vi "thermal PRF check by PID.vi"(0 "meas_setting":T2={"measSetId"=6949, "measSetComments"="Orchid", "probeId"=141.0, "beamstyleIndex"=0, "txFrequencyHz"=3636400.0, "focusRangeCm"=8.0, "maxTxVoltageVolt"=100.0, "ceilTxVoltageVolt"=80.0, "profTxVoltageVolt"=62.0, "totalVoltagePt"=20, "numMeasVoltage"=12, "numTxElements"=118, "txpgWaveformStyle"=2, "numTxCycles"=4.0, "elevAperIndex"=0, "zStartDistCm"=1.5, "zMeasNum"=80, "IsTxAperModulationEn"=0, "DTxFreqIndex"=0, "VTxIndex"=0, "IsCPAEn"=0, "SysPulserSelA"=0, "TxPulseRleA"=""} {"zStartDistCm" format="%.2f"; "numTxCycles" format="%.1f"; "profTxVoltageVolt" format="%#_1g"; "ceilTxVoltageVolt" format="%.2f"; "maxTxVoltageVolt" format="%.2f"; "focusRangeCm" format="%.1f"; "txFrequencyHz" format="%.2f"}, 1 "PRF":dbl format="%.2f", 2 "Measurement Type":enum32{"Volt", "SA"}(radio), 5 "TCP from Orchid in":refnum<k5>, 9 "tcp time out":dbl format="%.2f", 11 "voltage":dbl format="%.2f", 12 "Comment(SN)":string) -> (4 "PRF":dbl format="%#.2f", 10 "Command \nVerify":bool, 15 "Error(Volt & PRF)":bool)   [LabVIEW 2016]
uses:
  type def/measSetting.ctl
  user/GrobaLimitVoltage.vi
  Thermal_type.vi
  <vilib>/Instr/_visa.llb/VISA Configure Serial Port (Instr).vi
  Instance          12 30Saved   thermal PRF&Volt check .vi
  Instance          18 30Saved   thermal PRF&Volt check .vi
panel:
  out "error out 4":errorcluster
  out "error out 3":errorcluster
  in  "취소 버튼":bool
  out "경과시간(S)":string caption="경과 시간 텍스트"
  out "TempRise":dbl format="%.2f"
  out "Probe":dbl format="%.2f"
  out "Ambient":dbl format="%.2f"
  out "웨이브폼 차트":dbl(graph)
  out "경과시간":dbl caption="경과 시간(초)" format="%#.1g"
  out "Finish Time":string="7/29/2002  5:00 PM"
  out "Target  Temp.":i32
  out "Ambient":dbl
  out "Transducer":dbl
  out "error out 2":errorcluster
  out "Initial PRF":dbl format="%.2f"
  out "Current Voltage":dbl format="%.2f"
  out "Output Limit Voltage":i16
  out "Start Time":string="7/29/2002  5:00 PM"
  in  "stop 3":bool
  in  "meas_temparature_result":T1={"probeId"=10.0, "comments"="4C1 WCS", "tempSSId"=2, "measDate"="", "measSetNum"=1, "roomTempC"=0.0, "pulseVoltage"=80.0, "temperatureC"=0.0, "numTxCycles"=3.0, "numTxElements"=22, "txFrequencyHz"=3636400.0, "elevAperIndex"=0, "isTxAperModulationEn"=0, "txpgWaveformStyle"=0, "pulseRepetRate"=610.0, "scanRange"=0.0, "tempSetId"=0, "IsSCW"=0, "VTxIndex"=0} {"temperatureC" format="%.2f"; "scanRange" format="%.2f"; "pulseRepetRate" format="%.6f"; "roomTempC" format="%.2f"; "numTxCycles" format="%#_1f"}
  out "Result":string
  in  "file path":path=path "C:/temp log data/TempResultData"
  out "Waveform Chart":cluster{dbl, dbl, i32, i32}(graph)
  out "error out":errorcluster
  # "To find PRF by PID"
  # "Cooling"
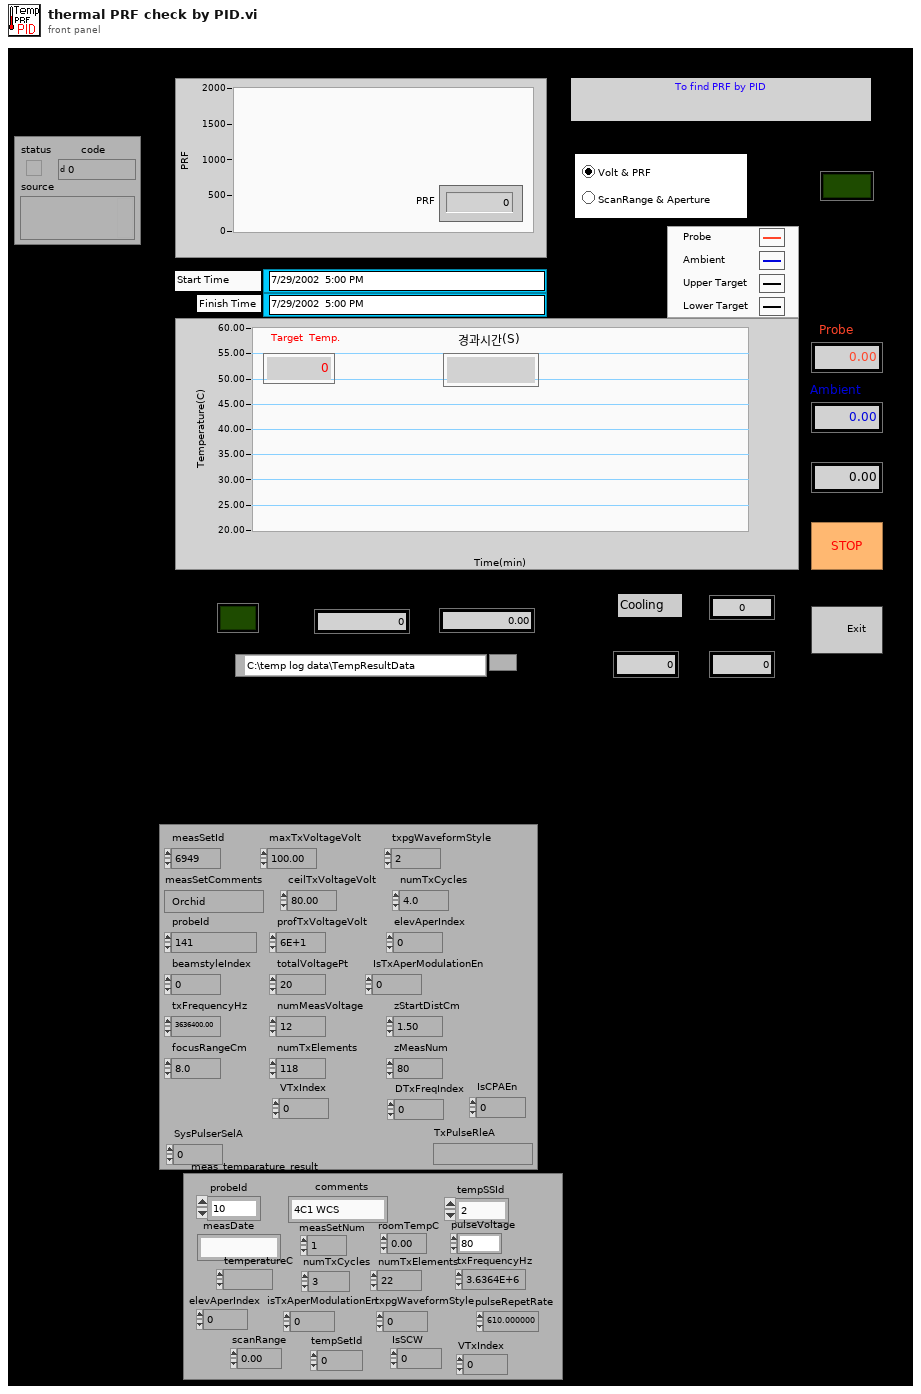
[diagram p1: front panel]
types:
  T1 = cluster{"probeId":sgl, "comments":string, "tempSSId":i16, "measDate":string, "measSetNum":i16, "roomTempC":sgl, "pulseVoltage":dbl, "temperatureC":ext, "numTxCycles":dbl, "numTxElements":i16, "txFrequencyHz":dbl, "elevAperIndex":i16, "isTxAperModulationEn":i16, "txpgWaveformStyle":i16, "pulseRepetRate":dbl, "scanRange":dbl, "tempSetId":i16, "IsSCW":i16, "VTxIndex":i16}
  T2 = typedef "measSetting.ctl" = cluster{"measSetId":i32, "measSetComments":string, "probeId":sgl, "beamstyleIndex":i16, "txFrequencyHz":sgl, "focusRangeCm":sgl, "maxTxVoltageVolt":sgl, "ceilTxVoltageVolt":sgl, "profTxVoltageVolt":dbl, "totalVoltagePt":i8, "numMeasVoltage":i8, "numTxElements":i16, "txpgWaveformStyle":i8, "numTxCycles":sgl, "elevAperIndex":i8, "zStartDistCm":sgl, "zMeasNum":i8, "IsTxAperModulationEn":i8, "DTxFreqIndex":i16, "VTxIndex":i8, "IsCPAEn":i16, "SysPulserSelA":i16, "TxPulseRleA":string}
  T3 = enum16{"open", "open or create", "create or replace", "create", "open (read only)"}
  T4 = cluster{"Output probe":dbl, "Output ambient":dbl, i32, i32}
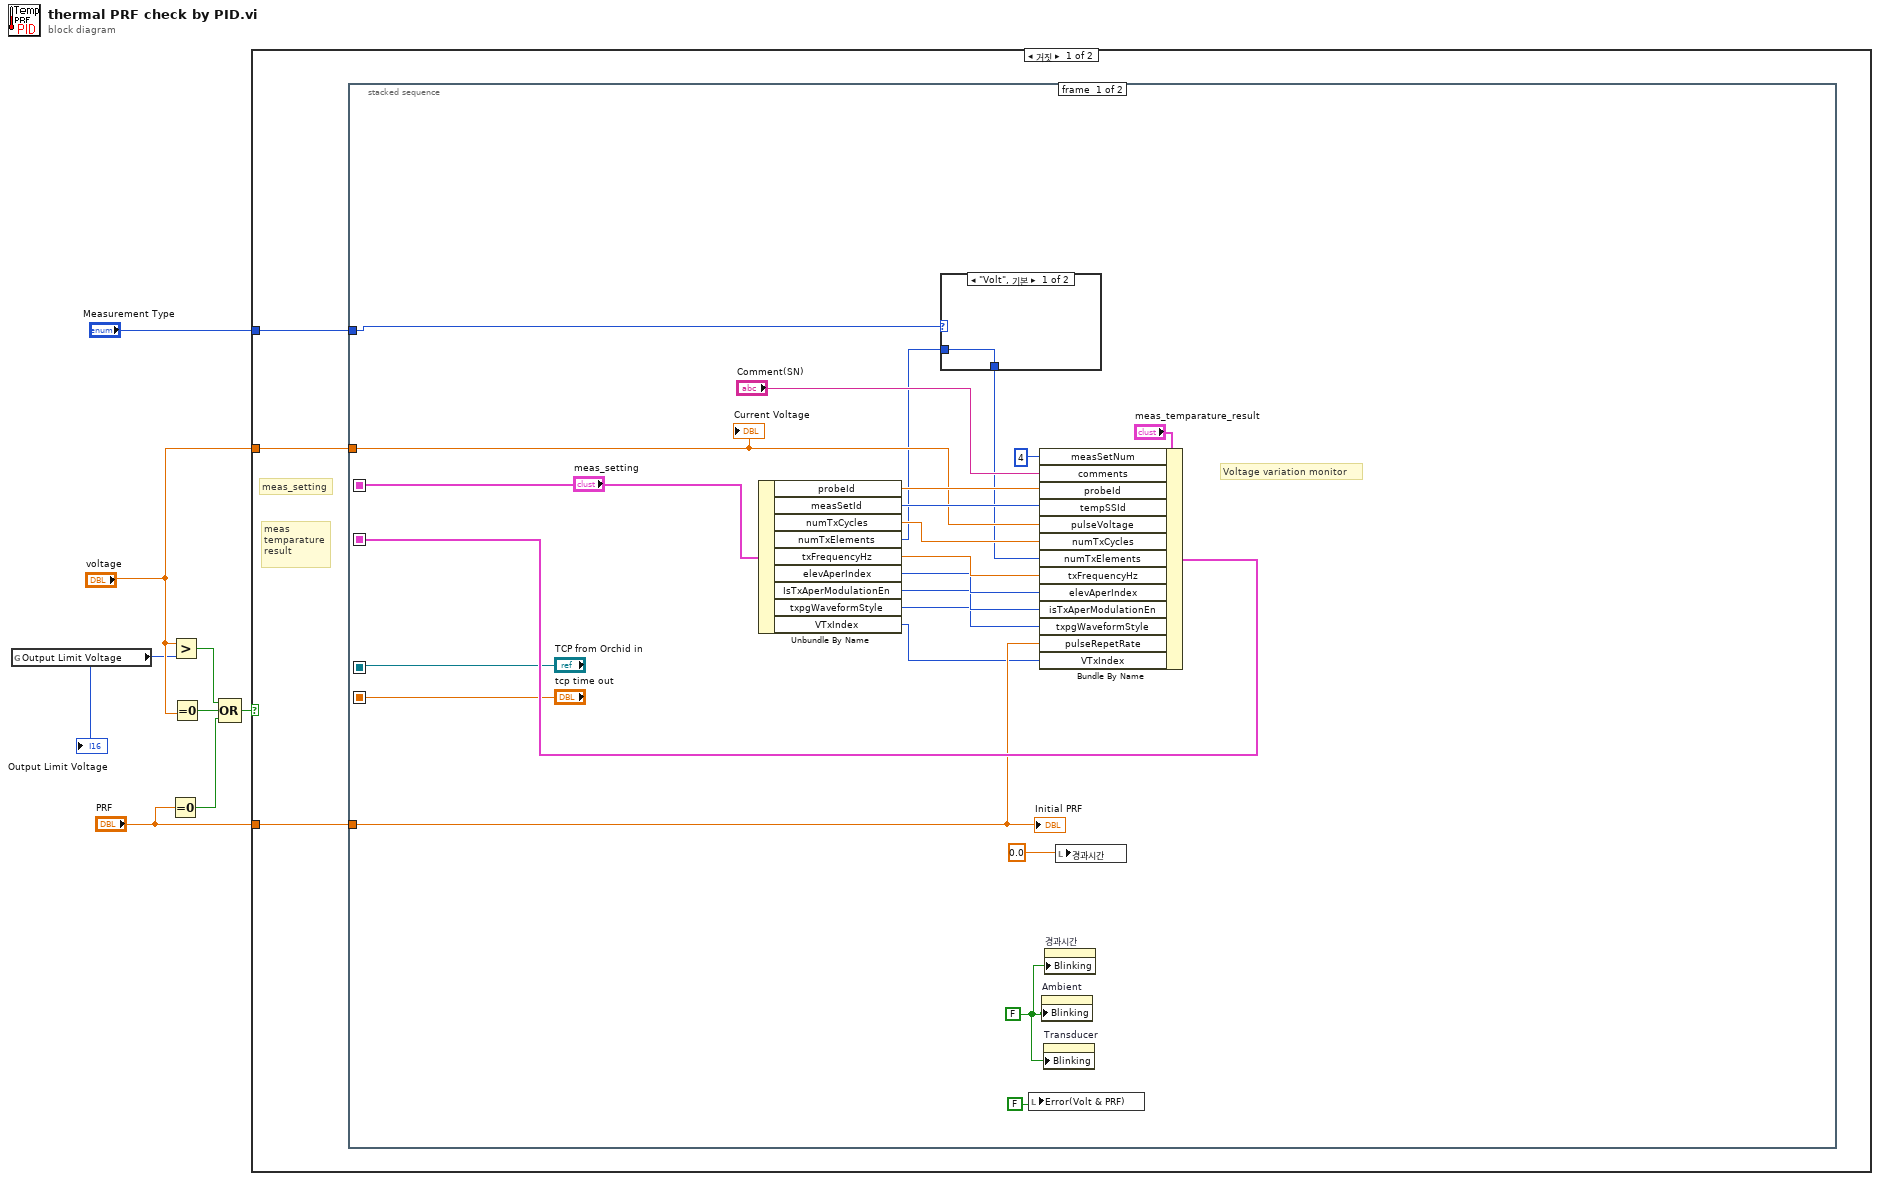
[diagram p0: block diagram]
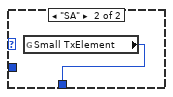
[diagram p2: hidden frame]
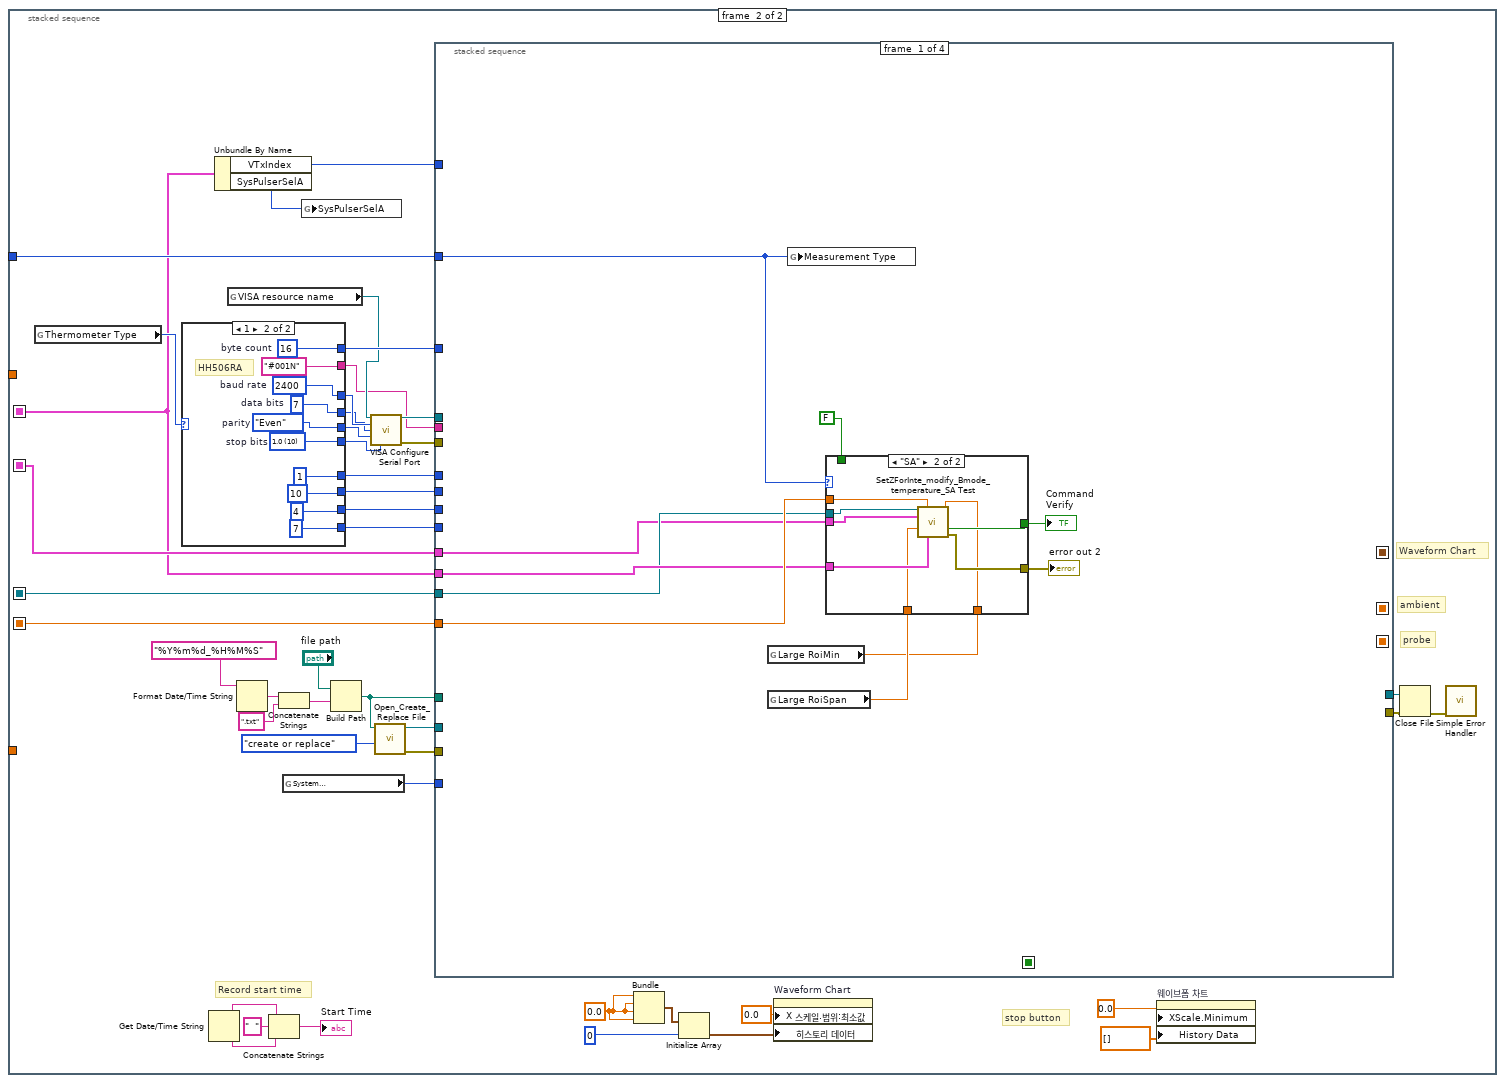
[diagram p3: hidden frame]
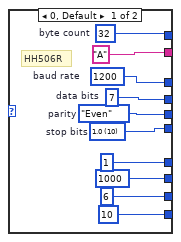
[diagram p4: hidden frame]
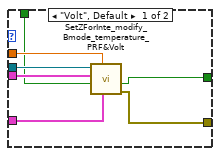
[diagram p5: hidden frame]
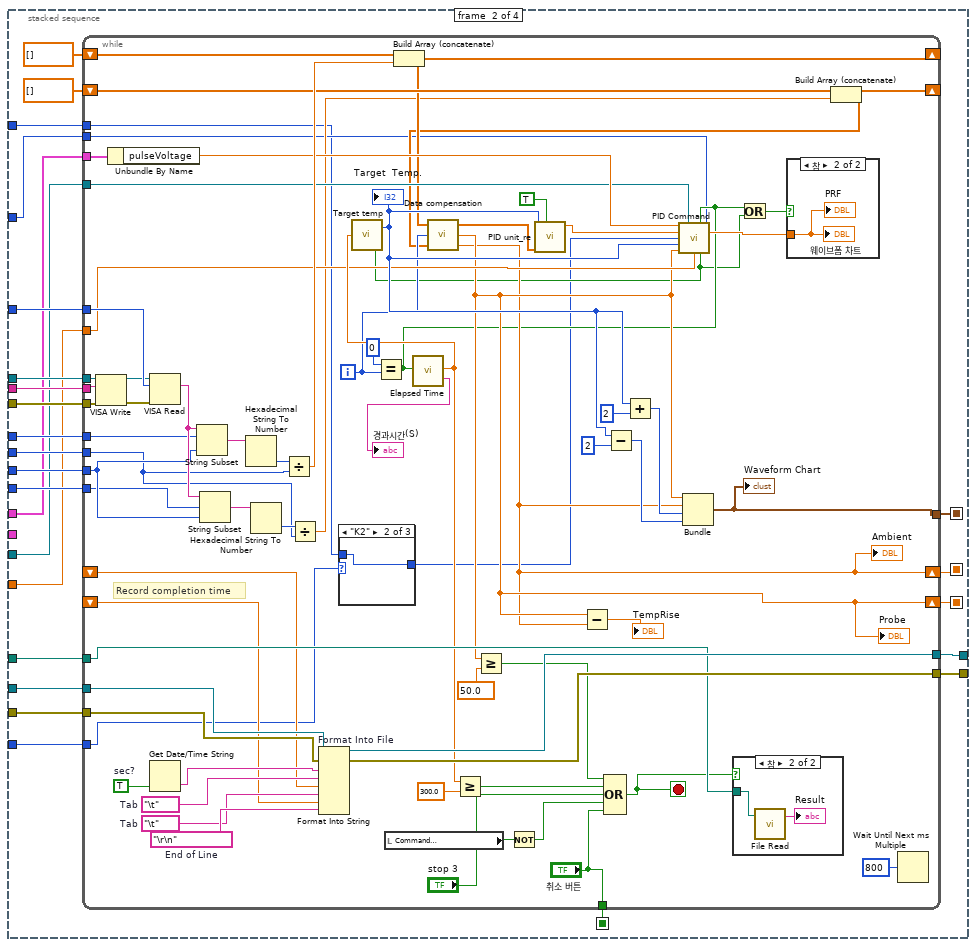
[diagram p6: hidden frame]
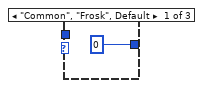
[diagram p7: hidden frame]
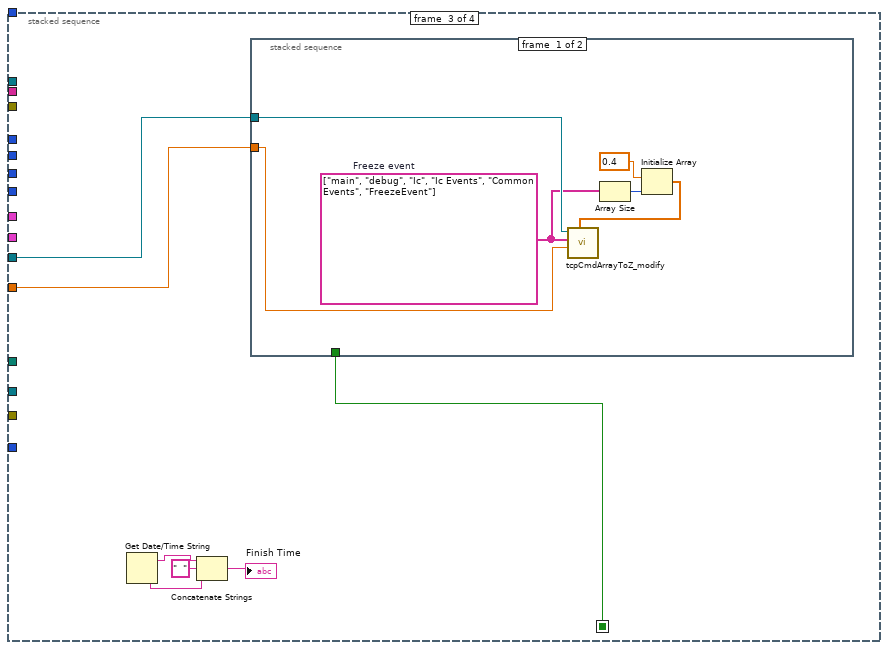
[diagram p11: hidden frame]
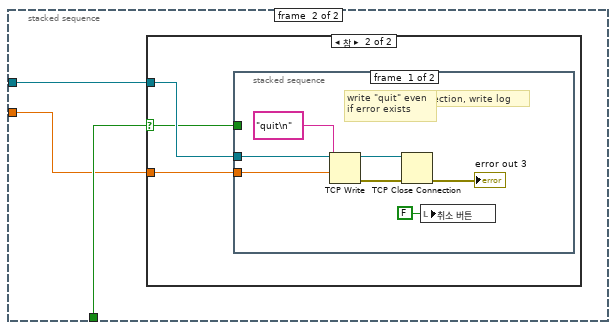
[diagram p12: hidden frame]
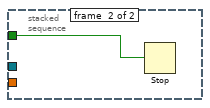
[diagram p14: hidden frame]
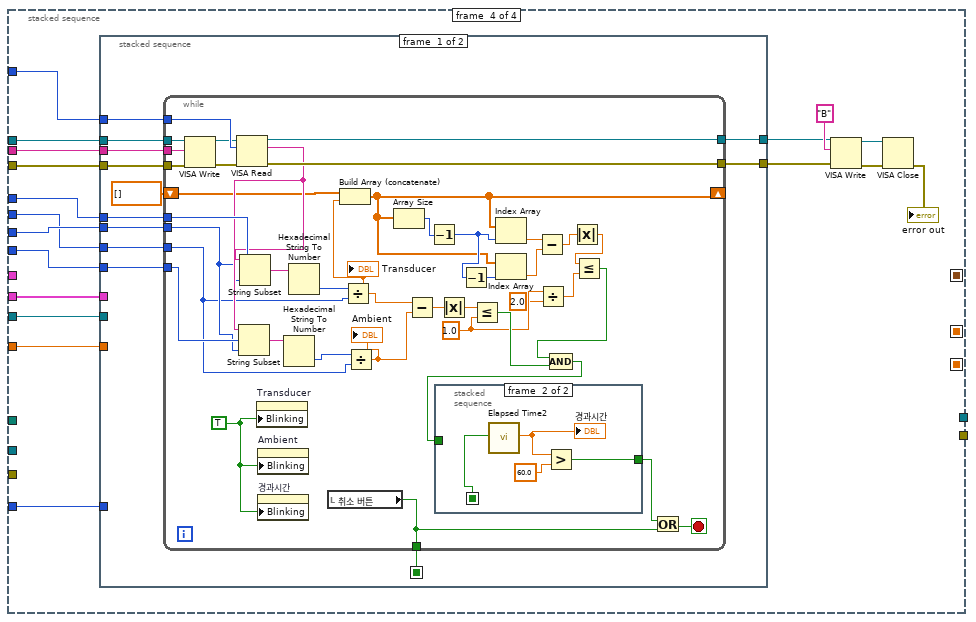
[diagram p15: hidden frame]
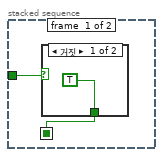
[diagram p16: hidden frame]
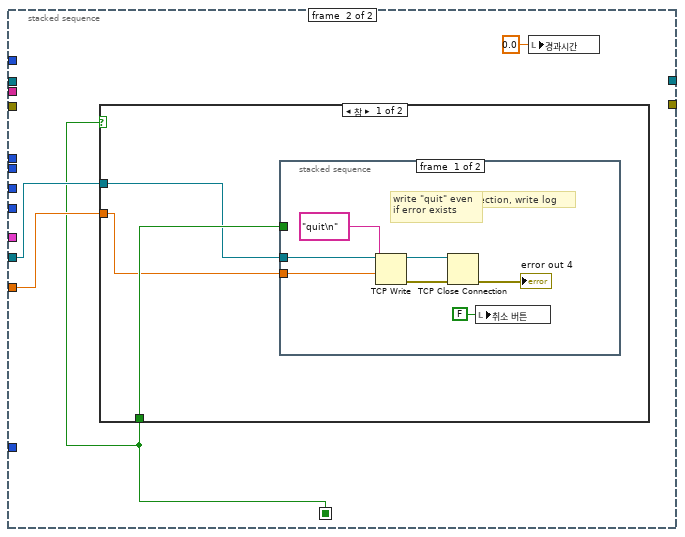
[diagram p18: hidden frame]
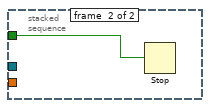
[diagram p19: hidden frame]
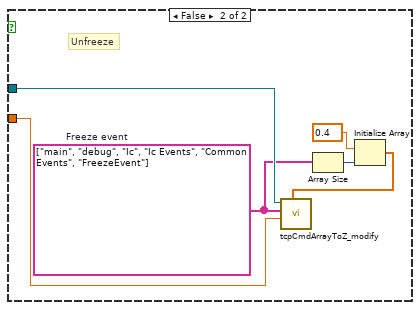
[diagram p20: hidden frame]
diagram:
  n1 = global read "GrobaLimitVoltage.vi" "Output Limit Voltage"() -> (w7:i16)
  "Output Limit Voltage" <- w7
  n2 = Equal To 0?(x="PRF") -> (x = 0?=w2:bool)
  n3 = Greater?(x="voltage", y=w7) -> (0:w6:bool)
  n4 = Equal To 0?(x="voltage") -> (x = 0?=w5:bool)
  n5 = Compound Arithmetic op=OR(w6, w5, w2) -> (w4:bool)
  n6 = case shown="거짓" w4 {
    tunnel: "voltage" -> [w11 _]
    tunnel: "PRF" -> [w10 _]
    tunnel: "Measurement Type" -> [w9 _]
    frame False {
      # "meas\ntemparature\nresult"
      # "meas_setting"
      n7 = stacked-sequence {
        seq-local: ["meas_setting" _] -> [_ w38]
        seq-local: [w24 _] -> [_ w69]
        seq-local: ["TCP from Orchid in" _] -> [_ w68]
        seq-local: ["tcp time out" _] -> [_ w67]
        tunnel: w11 -> [w22 _]
        tunnel: w10 -> [w21 _]
        tunnel: w9 -> [w15 w41]
        frame #0 {
          w17 = FALSE ("점멸")
          # "Voltage variation monitor"
          n8 = Unbundle By Name("meas_setting") -> ("probeId"=w31:sgl, "measSetId"=w30:i32, "numTxCycles"=w29:sgl, "numTxElements"=w13:i16, "txFrequencyHz"=w28:sgl, "elevAperIndex"=w27:i8, "IsTxAperModulationEn"=w26:i8, "txpgWaveformStyle"=w25:i8, "VTxIndex"=w12:i8)
          n9 = case shown="\"Volt\", 기본" w15 {
            tunnel: [w35 w36] -> w14
            tunnel: w13 -> [w35 _]
            frame "Volt", Default {
            }
            frame "SA" {
              n10 = global read "Thermal_type.vi" "Small TxElement"() -> (w36:i32)
            }
          }
          n11 = local write "Error(Volt & PRF)"(FALSE) -> ()
          n12 = Bundle By Name(cluster="meas_temparature_result", "measSetNum"=i16 4, "comments"="Comment(SN)", "probeId"=w31, "tempSSId"=w30, "pulseVoltage"=w22, "numTxCycles"=w29, "numTxElements"=w14, "txFrequencyHz"=w28, "elevAperIndex"=w27, "isTxAperModulationEn"=w26, "txpgWaveformStyle"=w25, "pulseRepetRate"=w21, "VTxIndex"=w12) -> (w24:T1)
          n13 = property on="Ambient" class="DigNum (엄격한)"("Blinking"=w17) -> ()  [unwired: 2 in, 2 out]
          n14 = property on="Transducer" class="DigNum (엄격한)"("Blinking"=w17) -> ()  [unwired: 2 in, 2 out]
          n15 = property on="경과시간" class="DigNum (엄격한)"("Blinking"=w17) -> ()  [unwired: 2 in, 2 out]
          n16 = local write "경과시간"(0.0 ("Elapsed Time (s)")) -> ()
          "Current Voltage" <- w22
          "Initial PRF" <- w21
        }
        frame #1 {
          w44 = 0.0
          # "Record start time"
          # "Waveform Chart"
          # "ambient"
          # "probe"
          # "stop button"
          n17 = global read "Thermal_type.vi" "Thermometer Type"() -> (w59:u16)
          n18 = case shown="1" w59 {
            tunnel: [w91 w100] -> w57
            tunnel: [w90 w99] -> w56
            tunnel: [w89 w98] -> w55
            tunnel: ["A" ("write buffer (\"\")") "#001N" ("write buffer (\"\")")] -> w46
            tunnel: [w87 w97] -> w54
            tunnel: [10 ("offset (0)") 7 ("offset (0)")] -> w51
            tunnel: [6 ("length (rest)") 4 ("length (rest)")] -> w52
            tunnel: [u32 1000 ("y") u32 10 ("y")] -> w50
            tunnel: [1 ("offset (0)") 1 ("offset (0)")] -> w53
            tunnel: [w82 w92] -> w58
            frame 0, Default {
              w82 = u32 32  # byte count
              w87 = u16 10 items=["1.0"=10, "1.5"=15, "2.0"=20]  # stop bits
              w89 = enum16{"None", "Odd", "Even", "Mark", "Space"}."Even"  # parity
              w90 = u16 7  # data bits
              w91 = u32 1200  # baud rate
              # "HH506R"
            }
            frame 1 {
              w92 = u32 16  # byte count
              w97 = u16 10 items=["1.0"=10, "1.5"=15, "2.0"=20]  # stop bits
              w98 = enum16{"None", "Odd", "Even", "Mark", "Space"}."Even"  # parity
              w99 = u16 7  # data bits
              w100 = u32 2400  # baud rate
              # "HH506RA"
            }
          }
          n19 = Get Date/Time String() -> (date string=w65:string, time string=w63:string)  [unwired: 3 in]
          n20 = Unbundle By Name(w38) -> ("VTxIndex"=w40:i8, "SysPulserSelA"=w37:i16)
          n21 = global read "Thermal_type.vi" "VISA resource name"() -> (w49:refnum<visa-resource-name>)
          n22 = Format Date/Time String(time format string (%c)="%Y%m%d_%H%M%S") -> (date/time string=w62:string)  [unwired: 2 in]
          n23 = Concatenate Strings(w65, "  ", w63) -> (→"Start Time":string)
          n24 = Concatenate Strings(w62, ".txt" ("string")) -> (w70:string)
          n25 = global read "Thermal_type.vi" "System \nSelection"() -> (w39:enum32{"Common", "Frosk", "Griffin", "K2"})
          n26 = global write "Thermal_type.vi" "SysPulserSelA"(w37) -> ()
          n27 = Build Path(base path="file path", name or relative path=w70) -> (appended path=w71:path)
          n28 = call-poly "VISA Configure Serial Port"("VISA resource name"=w49, "baud rate (9600)"=w57, "data bits (8)"=w56, "parity (0:none)"=w55, "stop bits (10: 1 bit)"=w54) -> ("VISA resource name out"=w48:refnum<visa-resource-name>, "error out"=w47:errorcluster)  [unwired: 9 in]
          n29 = call <vilib>:"Open_Create_Replace File.vi"("function (open:0)"=T3."create or replace", "file path"=w71) -> ("error out"=w80:errorcluster, "refnum"=w81:refnum<file>)  [unwired: 6 in, 2 out]
          n30 = stacked-sequence {
            seq-local: [_ w146 _ _] -> [_ _ _ _]
            seq-local: [_ w145 _ _] -> [_ _ _ _]
            seq-local: [_ w144 _ _] -> [_ _ _ _]
            seq-local: [_ w127 _ _] -> [_ _ w229 _]
            tunnel: w81 -> [_ w151 _ _]
            tunnel: w80 -> [_ w150 _ _]
            tunnel: [_ w149 _ _] -> w78
            tunnel: [_ w148 _ _] -> w76
            tunnel: w71 -> [_ w147 _ _]
            tunnel: w69 -> [w108 w132 _ _]
            tunnel: w68 -> [w109 w135 w231 w267]
            tunnel: w67 -> [w111 w134 w230 w266]
            tunnel: w38 -> [w110 _ _ w257]
            tunnel: w58 -> [_ w143 _ w262]
            tunnel: w53 -> [_ w142 _ w265]
            tunnel: w52 -> [_ w141 _ w264]
            tunnel: w51 -> [_ w140 _ w258]
            tunnel: w50 -> [_ w139 _ w263]
            tunnel: w48 -> [_ w138 _ w261]
            tunnel: w47 -> [_ w137 _ w260]
            tunnel: w46 -> [_ w136 _ w259]
            tunnel: w41 -> [w105 w128 _ _]
            tunnel: w40 -> [_ w130 _ _]
            tunnel: w39 -> [_ w129 _ w256]
            frame #0 {
              n31 = global read "Thermal_type.vi" "Large RoiMin"() -> (w103:dbl)
              n32 = global read "Thermal_type.vi" "Large RoiSpan"() -> (w104:dbl)
              n33 = global write "Thermal_type.vi" "Measurement Type"(w105) -> ()
              n34 = case shown="\"SA\"" w105 {
                tunnel: w111 -> [w118 w123]
                tunnel: w110 -> [w117 w125]
                tunnel: w109 -> [w116 w126]
                tunnel: w108 -> [w115 w124]
                tunnel: [w114 w122] -> w107
                tunnel: [w113 w121] -> w106
                tunnel: w104 -> [_ w120]
                tunnel: w103 -> [_ w119]
                tunnel: FALSE ("CW") -> [w112 _]
                frame "Volt", Default {
                  n35 = call "SetZForInte_modify_Bmode_temperature_PRF&Volt.vi"("meas_setting"=w117, "timeout (ms)"=w118, "CW"=w112, "meas_temparature_Input"=w115, "TCP from Orchid in"=w116) -> ("error out"=w113:errorcluster, "veri_P/F"=w114:bool)  [unwired: 3 in, 2 out]
                }
                frame "SA" {
                  n36 = call "SetZForInte_modify_Bmode_temperature_SA Test.vi"("TCP from Orchid in"=w126, "timeout (ms)"=w123, "RoiLaterMin"=w119, "meas_temparature_Input"=w124, "RoiLateralSpan"=w120, "meas_setting"=w125) -> ("veri_P/F"=w122:bool, "error out"=w121:errorcluster)  [unwired: 6 in, 2 out]
                }
              }
              "Command \nVerify" <- w107
              "error out 2" <- w106
            }
            frame #1 {
              n37 = while {
                shift-right: [w162] -> w146
                shift-left: _ -> [w203]
                shift-right: [w163] -> w145
                shift-left: _ -> [w190]
                tunnel: w151 -> [w219]
                tunnel: w150 -> [w218]
                tunnel: [w217] -> w148
                tunnel: [w216] -> w149
                tunnel: w147 -> [w212]
                tunnel: [w188] -> w144
                tunnel: w143 -> [w200]
                tunnel: w142 -> [w199]
                tunnel: w141 -> [w198]
                tunnel: w140 -> [w197]
                tunnel: w139 -> [w196]
                tunnel: w138 -> [w195]
                tunnel: w137 -> [w194]
                tunnel: w136 -> [w191]
                tunnel: w135 -> [w170]
                tunnel: w134 -> [w171]
                shift-right: [w168] -> _
                shift-left: dbl[] [] -> [w187]
                tunnel: w132 -> [w184]
                shift-right: [w165] -> _
                shift-left: dbl[] [] -> [w169]
                tunnel: w130 -> [w152]
                tunnel: w129 -> [w156]
                tunnel: w128 -> [w154]
                tunnel: ["취소 버튼"] -> w127
                i -> [w166]
                stop <- w210 stop-if-true
                w214 = "\t"  # Tab
                w215 = "\r\n"  # End of Line
                w220 = "\t"  # Tab
                w221 = TRUE  # sec?
                # "Record completion time"
                n38 = VISA Write(VISA resource name=w195, write buffer=w191, error in (no error)=w194) -> (VISA resource name out=w193:refnum<visa-resource-name>, error out=w192:errorcluster)  [unwired: 1 out]
                n39 = Unbundle By Name(w184) -> ("pulseVoltage"=w174:dbl)
                n40 = VISA Read(VISA resource name=w193, byte count=w200, error in (no error)=w192) -> (read buffer=w202:string)  [unwired: 3 out]
                n41 = Get Date/Time String(want seconds? (F)=w221) -> (time string=w213:string)  [unwired: 2 in, 1 out]
                n42 = String Subset(string=w202, offset (0)=w199, length (rest)=w198) -> (substring=w207:string)
                n43 = String Subset(string=w202, offset (0)=w197, length (rest)=w198) -> (substring=w205:string)
                n44 = Hexadecimal String To Number(string=w207) -> (number=w206:u32)  [unwired: 2 in, 1 out]
                n45 = Hexadecimal String To Number(string=w205) -> (number=w204:u32)  [unwired: 2 in, 1 out]
                n46 = Divide(x=w206, y=w196) -> (x/y=w175:dbl)
                n47 = Divide(x=w204, y=w196) -> (x/y=w164:dbl)
                n48 = Format Into String "Format Into File"(initial string=w219, error in=w218, w213, w220, w203, w214, w190, w215) -> (resulting string=w217:refnum<file>, error out=w216:errorcluster)  [unwired: 1 in]
                n49 = case shown="\"K2\"" w156 {
                  tunnel: [0 w224 w225] -> w155
                  tunnel: w152 -> [_ w224 w225]
                  frame "Common", "Frosk", Default {
                  }
                  frame "K2" {
                  }
                  frame "Griffin" {
                  }
                }
                n50 = Equal?(x=0, y=w166) -> (x = y?=w159:bool)
                n51 = local read "Command \nVerify"() -> (w186:bool)
                n52 = Build Array (concatenate)(w187, w175) -> (w168:dbl[])
                n53 = call "Elapsed Time"("Reset"=w159) -> ("Elapsed Time (s)"=w181:dbl, "Elapsed Time Text"=→"경과시간(S)":string)  [unwired: 11 in, 6 out]
                n54 = call "Target temp.vi"("elapsed time"=w181) -> ("Target temperature"=w172:i32, "control"=w158:bool)
                "Target  Temp." <- w172
                n55 = Greater Or Equal?(x=w181, y=300.0) -> (x >= y?=w182:bool)
                n56 = Not(x=w186) -> (.not. x?=w185:bool)
                n57 = Subtract(x=w172, y=2) -> (x-y=w176:i32)
                n58 = Add(x=w172, y=2) -> (x+y=w178:i32)
                n59 = Or(x=w159, y=w158) -> (x .or. y?=w160:bool)
                n60 = Build Array (concatenate)(w169, w164) -> (w165:dbl[])
                n61 = call "Data compensation.vi"("Input ambient"=w165, "Index"=w166, "Input probe"=w168) -> ("Output ambient"=w162:dbl, "Output probe"=w163:dbl, "Output probe array"=w167:dbl[])
                "Ambient" <- w162
                "Probe" <- w163
                n62 = Greater Or Equal?(x=w163, y=50.0) -> (x >= y?=w209:bool)
                n63 = call "PID unit_re.vi"("PID"=TRUE, "현재 온도"=w167, "Target 온도"=w172) -> ("적정 PRF"=w173:dbl)  [unwired: 6 in]
                n64 = Subtract(x=w163, y=w162) -> (x-y=→"TempRise":dbl)
                n65 = Compound Arithmetic op=OR(w209, w182, "stop 3", w185, "취소 버튼") -> (w210:bool)
                n66 = call "PID Command.vi"("PulseVoltage"=w174, "TCP from Orchid in"=w170, "Starting index"=w159, "Measurement Type"=w154, "적정 PRF"=w173, "VTxIndex"=w155, "Target temp"=w172, "Probe temp"=w163, "tcp time out"=w171, "Control enable"=w158) -> ("PRF"=w161:dbl)  [unwired: 5 in]
                n67 = Bundle("Output probe"=w163, "Output ambient"=w162, w178, w176) -> (w188:T4)  [unwired: 1 in]
                "Waveform Chart" <- w188
                n68 = case shown="참" w210 {
                  tunnel: w212 -> [_ w227]
                  frame False {
                  }
                  frame True {
                    n69 = call "File Read.vi"("file path"=w227) -> ("data"=→"Result":string)  [unwired: 3 in]
                  }
                }
                n70 = case shown="참" w160 {
                  tunnel: w161 -> [_ w226]
                  frame False {
                  }
                  frame True {
                    "웨이브폼 차트" <- w226
                    "PRF" <- w226
                  }
                }
                n71 = Wait Until Next ms Multiple(millisecond multiple=u32 800 ("milliseconds to wait")) -> ()  [unwired: 1 out]
              }
            }
            frame #2 {
              n72 = Get Date/Time String() -> (date string=w232:string, time string=w235:string)  [unwired: 3 in]
              n73 = Concatenate Strings(w232, "  ", w235) -> (→"Finish Time":string)
              n74 = stacked-sequence {
                tunnel: w231 -> [w241 w243]
                tunnel: w230 -> [w240 w242]
                tunnel: w229 -> [_ w244]
                frame #0 {
                  w237 = string[] ["main", "debug", "Ic", "Ic Events", "Common Events", "FreezeEvent"]  # Freeze event
                  n75 = Array Size(array=w237) -> (size(s)=w239:i32)
                  n76 = Initialize Array(0.4 ("element"), w239) -> (w236:dbl[])
                  n77 = call "tcpCmdArrayToZ_modify.vi"("Delay (sec)"=w236, "Timeout (ms)"=w240, "Command array"=w237, "connection ID in"=w241) -> ()  [unwired: 3 in, 5 out]
                }
                frame #1 {
                  n78 = case shown="참" w244 {
                    selector: w244 -> [_ w245]
                    tunnel: w243 -> [_ w247]
                    tunnel: w242 -> [_ w246]
                    frame False {
                    }
                    frame True {
                      n79 = stacked-sequence {
                        tunnel: w247 -> [w250 _]
                        tunnel: w246 -> [w249 _]
                        tunnel: w245 -> [_ w255]
                        frame #0 {
                          # "Close telnet connection, write log"
                          # "write \"quit\" even\nif error exists"
                          n80 = TCP Write(connection ID=w250, data in="quit\n", 9:w249) -> (connection ID out=w251:refnum<k5>, error out=w253:errorcluster)  [unwired: 1 in, 1 out]
                          n81 = TCP Close Connection(connection ID=w251, error in (no error)=w253) -> (error out=→"error out 3":errorcluster)  [unwired: 1 in, 1 out]
                          n82 = local write "취소 버튼"(FALSE ("취소 버튼")) -> ()
                        }
                        frame #1 {
                          n83 = Stop(stop? (T)=w255) -> ()
                        }
                      }
                    }
                  }
                }
              }
            }
            frame #3 {
              n84 = stacked-sequence {
                seq-local: [w274 _] -> [_ w333]
                tunnel: [w285 _] -> w269
                tunnel: [w284 _] -> w268
                tunnel: w267 -> [_ w335]
                tunnel: w266 -> [_ w334]
                tunnel: w265 -> [w283 _]
                tunnel: w264 -> [w282 _]
                tunnel: w263 -> [w281 _]
                tunnel: w262 -> [w280 _]
                tunnel: w261 -> [w279 _]
                tunnel: w260 -> [w278 _]
                tunnel: w259 -> [w277 _]
                tunnel: w258 -> [w276 _]
                tunnel: w257 -> [_ _]
                tunnel: w256 -> [_ _]
                frame #0 {
                  n85 = while {
                    tunnel: [w323] -> w285
                    tunnel: [w322] -> w284
                    tunnel: w283 -> [w321]
                    tunnel: w282 -> [w312]
                    tunnel: w281 -> [w309]
                    tunnel: w280 -> [w320]
                    tunnel: w279 -> [w319]
                    tunnel: w278 -> [w317]
                    tunnel: w277 -> [w315]
                    tunnel: w276 -> [w314]
                    shift-right: [w299] -> _
                    shift-left: dbl[] [] -> [w304]
                    tunnel: [w286] -> w274
                    stop <- w288 stop-if-true
                    w289 = TRUE ("점멸")
                    w296 = 1.0 ("y")
                    n86 = VISA Write(VISA resource name=w319, write buffer=w315, error in (no error)=w317) -> (VISA resource name out=w318:refnum<visa-resource-name>, error out=w316:errorcluster)  [unwired: 1 out]
                    n87 = VISA Read(VISA resource name=w318, byte count=w320, error in (no error)=w316) -> (VISA resource name out=w323:refnum<visa-resource-name>, read buffer=w313:string, error out=w322:errorcluster)  [unwired: 1 out]
                    n88 = String Subset(string=w313, offset (0)=w314, length (rest)=w312) -> (substring=w311:string)
                    n89 = String Subset(string=w313, offset (0)=w321, length (rest)=w312) -> (substring=w325:string)
                    n90 = property on="Transducer" class="DigNum (엄격한)"("Blinking"=w289) -> ()  [unwired: 2 in, 2 out]
                    n91 = property on="Ambient" class="DigNum (엄격한)"("Blinking"=w289) -> ()  [unwired: 2 in, 2 out]
                    n92 = property on="경과시간" class="DigNum (엄격한)"("Blinking"=w289) -> ()  [unwired: 2 in, 2 out]
                    n93 = Hexadecimal String To Number(string=w311) -> (number=w310:u32)  [unwired: 2 in, 1 out]
                    n94 = Hexadecimal String To Number(string=w325) -> (number=w324:u32)  [unwired: 2 in, 1 out]
                    n95 = local read "취소 버튼"() -> (w286:bool)
                    n96 = Divide(x=w324, y=w309) -> (x/y=w305:dbl)
                    "Transducer" <- w305
                    n97 = Build Array (concatenate)(w304, w305) -> (w299:dbl[])
                    n98 = Divide(x=w310, y=w309) -> (x/y=w308:dbl)
                    "Ambient" <- w308
                    n99 = Array Size(array=w299) -> (size(s)=w303:i32)
                    n100 = Subtract(x=w305, y=w308) -> (x-y=w307:dbl)
                    n101 = Decrement(x=w303) -> (x-1=w301:i32)
                    n102 = Absolute Value(x=w307) -> (abs(x)=w306:dbl)
                    n103 = Decrement(x=w301) -> (x-1=w302:i32)
                    n104 = Less Or Equal?(x=w306, y=w296) -> (x <= y?=w297:bool)
                    n105 = Index Array(array=w299, index=w301) -> (element=w300:dbl)
                    n106 = Index Array(array=w299, index=w302) -> (element=w298:dbl)
                    n107 = Subtract(x=w300, y=w298) -> (x-y=w292:dbl)
                    n108 = Divide(x=w296, y=2.0) -> (x/y=w294:dbl)
                    n109 = Absolute Value(x=w292) -> (abs(x)=w291:dbl)
                    n110 = Less Or Equal?(x=w291, y=w294) -> (x <= y?=w293:bool)
                    n111 = Compound Arithmetic op=AND(w293, w297) -> (w290:bool)
                    n112 = stacked-sequence {
                      seq-local: [w326 _] -> [_ w329]
                      tunnel: w290 -> [w327 _]
                      tunnel: [_ w332] -> w287
                      frame #0 {
                        n113 = case shown="거짓" w327 {
                          tunnel: [TRUE _] -> w326
                          frame False {
                          }
                          frame True {
                          }
                        }
                      }
                      frame #1 {
                        n114 = call "Elapsed Time2"("Reset"=w329) -> ("Elapsed Time (s)"=w331:dbl)  [unwired: 11 in, 7 out]
                        "경과시간" <- w331
                        n115 = Greater?(x=w331, y=60.0) -> (0:w332:bool)
                      }
                    }
                    n116 = Or(x=w287, y=w286) -> (x .or. y?=w288:bool)
                  }
                }
                frame #1 {
                  n117 = case shown="참" w333 {
                    tunnel: w335 -> [w338 w353]
                    tunnel: w334 -> [w337 w352]
                    tunnel: w333 -> [w339 _]
                    frame True {
                      n118 = stacked-sequence {
                        tunnel: w338 -> [w342 _]
                        tunnel: w337 -> [w341 _]
                        tunnel: w339 -> [_ w347]
                        frame #0 {
                          # "Close telnet connection, write log"
                          # "write \"quit\" even\nif error exists"
                          n119 = TCP Write(connection ID=w342, data in="quit\n", 9:w341) -> (connection ID out=w343:refnum<k5>, error out=w345:errorcluster)  [unwired: 1 in, 1 out]
                          n120 = TCP Close Connection(connection ID=w343, error in (no error)=w345) -> (error out=→"error out 4":errorcluster)  [unwired: 1 in, 1 out]
                          n121 = local write "취소 버튼"(FALSE ("취소 버튼")) -> ()
                        }
                        frame #1 {
                          n122 = Stop(stop? (T)=w347) -> ()
                        }
                      }
                    }
                    frame False {
                      w349 = string[] ["main", "debug", "Ic", "Ic Events", "Common Events", "FreezeEvent"]  # Freeze event
                      # "Unfreeze"
                      n123 = Array Size(array=w349) -> (size(s)=w351:i32)
                      n124 = Initialize Array(0.4 ("element"), w351) -> (w348:dbl[])
                      n125 = call "tcpCmdArrayToZ_modify.vi"("Delay (sec)"=w348, "Timeout (ms)"=w352, "Command array"=w349, "connection ID in"=w353) -> ()  [unwired: 3 in, 5 out]
                    }
                  }
                  n126 = local write "경과시간"(0.0 ("경과시간")) -> ()
                }
              }
              n127 = VISA Write(VISA resource name=w269, write buffer="B" ("write buffer (\"\")"), error in (no error)=w268) -> (VISA resource name out=w273:refnum<visa-resource-name>, error out=w272:errorcluster)  [unwired: 1 out]
              n128 = VISA Close(VISA resource name=w273, error in (no error)=w272) -> (error out=→"error out":errorcluster)
            }
          }
          n129 = Bundle(w44, w44, w44, w44) -> (w73:cluster{dbl, dbl, dbl, dbl})  [unwired: 1 in]
          n130 = Initialize Array(w73, 0) -> (w45:cluster{dbl, dbl, dbl, dbl}[])
          n131 = property on="Waveform Chart" class="WFChart (엄격한)"("X 스케일.범위:최소값"=0.0 ("X Scale.Range:Minimum"), "히스토리 데이터"=w45) -> ()  [unwired: 2 in, 2 out]
          n132 = property on="웨이브폼 차트" class="WFChart (엄격한)"("XScale.Minimum"=0.0 ("X 스케일.범위:최소값"), "History Data"=dbl[] [] ("히스토리 데이터")) -> ()  [unwired: 2 in, 2 out]
          n133 = Close File(refnum=w76, error in=w78) -> (error out=w79:errorcluster)  [unwired: 1 out]
          n134 = call <vilib>:"Simple Error Handler.vi"("error in (no error)"=w79) -> ()  [unwired: 4 in, 5 out]
        }
      }
    }
    frame True {
      "Error(Volt & PRF)" <- TRUE
    }
  }
